vi "Rs232 Read.vi"(0 "VISA resource name":refnum<visa-resource-name> caption="VISA资源名称", 1 "baud rate (9600)":string, 2 "timeout (10sec)":u32=10000 caption="超时（10秒）", 3 "error in (no error)":errorcluster caption="错误输入（无错误）", 4 "Total Bytes":u32) -> (5 "Data Out":string, 6 "Error":errorcluster caption="错误输出")   [LabVIEW 2014]
uses:
  <vilib>/Instr/_visa.llb/VISA Configure Serial Port (Instr).vi
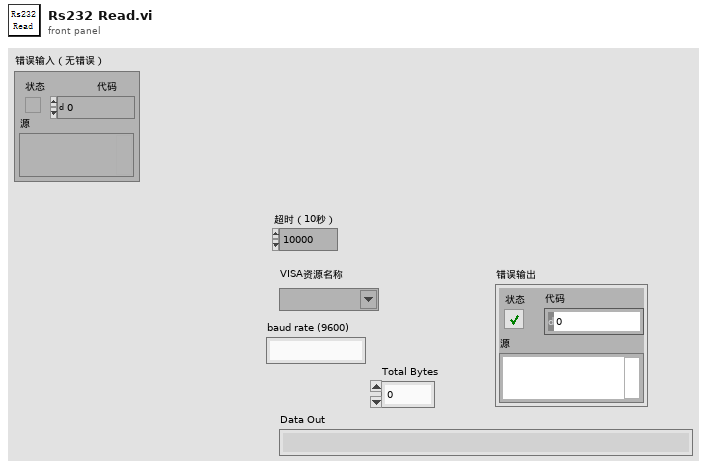
[diagram p1: front panel]
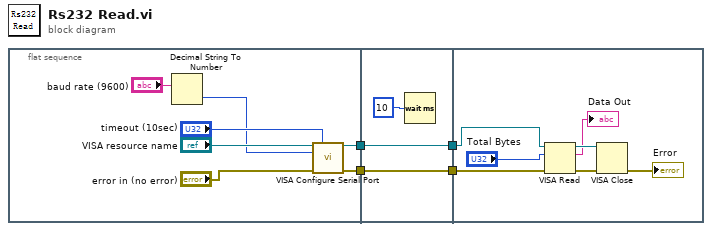
[diagram p0: block diagram]
diagram:
  n1 = flat-sequence {
    tunnel: [w9] -> w4
    tunnel: [w8] -> w3
    tunnel: [w13] -> w2
    tunnel: w4 -> [w13]
    tunnel: [w12] -> w1
    tunnel: w3 -> [w12]
    tunnel: w2 -> [w21]
    tunnel: w1 -> [w20]
    frame #0 {
      n2 = Decimal String To Number(string="baud rate (9600)") -> (number=w6:i32)  [unwired: 2 in, 1 out]
      n3 = call-poly "VISA Configure Serial Port"("VISA resource name"="VISA resource name", "timeout (10sec)"="timeout (10sec)", "baud rate (9600)"=w6, "error in (no error)"="error in (no error)") -> ("VISA resource name out"=w9:refnum<visa-resource-name>, "error out"=w8:errorcluster)  [unwired: 10 in]
    }
    frame #1 {
      n4 = Wait (ms)(milliseconds to wait=u32 10 ("等待时间（毫秒）")) -> ()  [unwired: 1 out]
    }
    frame #2 {
      n5 = VISA Read(VISA resource name=w21, byte count="Total Bytes", error in (no error)=w20) -> (VISA resource name out=w18:refnum<visa-resource-name>, read buffer=→"Data Out":string, error out=w17:errorcluster)  [unwired: 1 out]
      n6 = VISA Close(VISA resource name=w18, error in (no error)=w17) -> (error out=→"Error":errorcluster)
    }
  }
